vi "Launch TCP Nested Actors.vi"(8 "error in (no error)":errorcluster, 11 "Cfg Grandmaster in":refnum<class "Cfg Grandmaster.lvclass">) -> (0 "error out":errorcluster, 3 "Cfg Grandmaster out":refnum<class "Cfg Grandmaster.lvclass">)   [LabVIEW 2012, in "Configuration Grandmaster.lvlib" / "Cfg Grandmaster.lvclass"]
doc: "(<B>Filename</B>: Actor Framework.lvlib:Actor.lvclass:Pre Launch Init.vi)\n\nDefines behavior that occurs after the Launch Actor method is invoked but before the actor's Actor Core method begins running.\n\nThe Pre Launch Init method is guaranteed to finish before the Launch Actor method returns to its caller and before the actor itself receives any messages. Any references that the Pre Launch Init method obtains are guaranteed to have the same lifetime as the actor itself. Any errors that the Pre Launch Init method returns will abort the launch.\n\nBy default, this method does nothing. A descendant class may override it to define behavior."
uses:
  Cfg Grandmaster.lvclass
  <vilib>/ActorFramework/Actor/Actor.lvclass/Actor.ctl
  <vilib>/ActorFramework/Message Enqueuer/Message Enqueuer.lvclass/Message Enqueuer.ctl
  Cfg Grandmaster.lvclass/Cfg Grandmaster.ctl
  <vilib>/ActorFramework/Message Enqueuer/Init from Existing Queue.vi
  <vilib>/ActorFramework/Message Enqueuer/Enqueue.vi
  <vilib>/ActorFramework/Message Priority Queue/Priority Enqueue.vi
  <vilib>/ActorFramework/Message Enqueuer/Message Enqueuer.lvclass
  TCP Server/TCP Reader Messages/Listen Msg/Reader Listen Msg.lvclass
  TCP Server/TCP Writer Messages/Writer Listen Msg/Writer Listen Msg.lvclass
  <vilib>/ActorFramework/Actor/Actor.lvclass
  TCP Server/Class TCP Reader/TCP Reader.lvclass
  TCP Server/Class TCP Writer/TCP Writer.lvclass
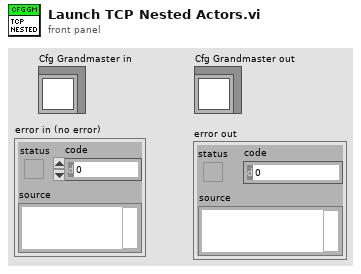
[diagram p1: front panel]
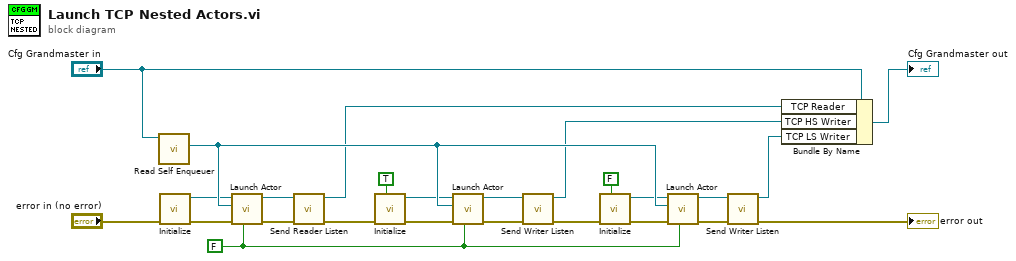
[diagram p0: block diagram]
diagram:
  w9 = FALSE ("Open Actor Core front panel? (F)")
  n1 = call <vilib>:"Read Self Enqueuer.vi"("Actor"="Cfg Grandmaster in") -> ("Self Enqueuer"=w25:refnum<class "Message Enqueuer.lvclass">)  [unwired: 10 in]
  n2 = call "Initialize.vi"("error in (no error)"="error in (no error)") -> ("error out"=w23:errorcluster, "TCP Reader out"=w24:refnum<class "TCP Reader.lvclass">)  [unwired: 9 in]
  n3 = call <vilib>:"Launch Actor.vi"("Open Actor Core front panel? (F)"=w9, "error in (no error)"=w23, "Actor-to-Caller Enqueuer"=w25, "Actor"=w24) -> ("error out"=w18:errorcluster, "Caller-To-Actor Enqueuer"=w17:refnum<class "Message Enqueuer.lvclass">)  [unwired: 6 in]
  n4 = call "Send Reader Listen.vi"("error in (no error)"=w18, "Message Enqueuer"=w17) -> ("error out"=w8:errorcluster, "Message Enqueuer out"=w4:refnum<class "Message Enqueuer.lvclass">)  [unwired: 8 in]
  n5 = call "Initialize.vi"("HS (T) / LS (F)"=TRUE, "error in (no error)"=w8) -> ("error out"=w21:errorcluster, "TCP Writer out"=w22:refnum<class "TCP Writer.lvclass">)  [unwired: 8 in]
  n6 = call <vilib>:"Launch Actor.vi"("Open Actor Core front panel? (F)"=w9, "error in (no error)"=w21, "Actor-to-Caller Enqueuer"=w25, "Actor"=w22) -> ("error out"=w15:errorcluster, "Caller-To-Actor Enqueuer"=w16:refnum<class "Message Enqueuer.lvclass">)  [unwired: 6 in]
  n7 = call "Send Writer Listen.vi"("error in (no error)"=w15, "Message Enqueuer"=w16) -> ("error out"=w7:errorcluster, "Message Enqueuer out"=w3:refnum<class "Message Enqueuer.lvclass">)  [unwired: 8 in]
  n8 = call "Initialize.vi"("HS (T) / LS (F)"=FALSE, "error in (no error)"=w7) -> ("error out"=w20:errorcluster, "TCP Writer out"=w19:refnum<class "TCP Writer.lvclass">)  [unwired: 8 in]
  n9 = call <vilib>:"Launch Actor.vi"("Open Actor Core front panel? (F)"=w9, "error in (no error)"=w20, "Actor-to-Caller Enqueuer"=w25, "Actor"=w19) -> ("error out"=w13:errorcluster, "Caller-To-Actor Enqueuer"=w14:refnum<class "Message Enqueuer.lvclass">)  [unwired: 6 in]
  n10 = call "Send Writer Listen.vi"("error in (no error)"=w13, "Message Enqueuer"=w14) -> ("error out"=→"error out":errorcluster, "Message Enqueuer out"=w2:refnum<class "Message Enqueuer.lvclass">)  [unwired: 8 in]
  n11 = Bundle By Name(cluster="Cfg Grandmaster in", "TCP Reader"=w4, "TCP HS Writer"=w3, "TCP LS Writer"=w2) -> (→"Cfg Grandmaster out":refnum<class "Cfg Grandmaster.lvclass">)
